vi "TEST - Delete Recursive (Read-Only).vi"(8 "error in (no error)":errorcluster) -> (0 "error out":errorcluster, 2 "pass":bool)   [LabVIEW 2020]
uses:
  source/library/File Exists/File Exists - Scalar.vi
  <userlib>/_OpenG.lib/error/error.llb/openg_error.lvlib
  source/library/openg_file.lvlib
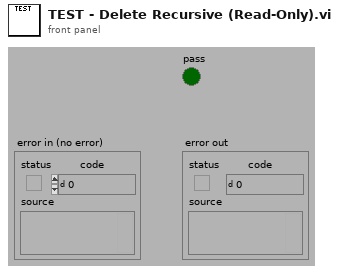
[diagram p1: front panel]
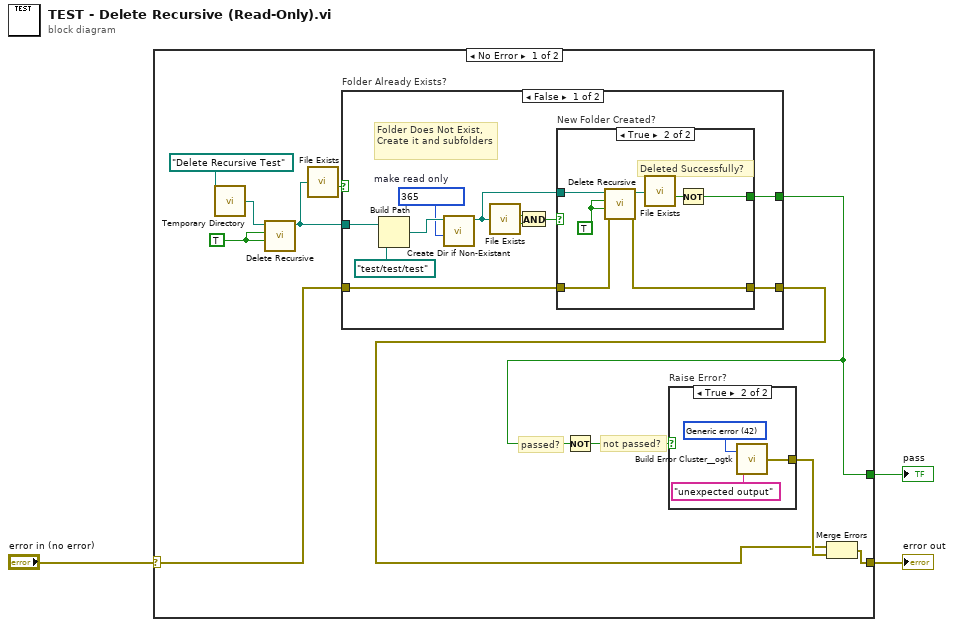
[diagram p0: block diagram]
diagram:
  n1 = case shown="No Error" "error in (no error)" {
    selector: "error in (no error)" -> [w4 w38]
    tunnel: [w5 _] -> w3
    tunnel: [w14 w38] -> w1
    frame No Error {
      w9 = TRUE ("Ignore Read-Only? (FALSE)")
      # "not passed?"
      # "passed?"
      n2 = call "Temporary Directory.vi"("Relative path (.)"=path "Delete Recursive Test") -> ("Temporary Directory (+ Relative)"=w10:path)
      n3 = call "Delete Recursive.vi"("Ignore Read-Only? (FALSE)"=w9, "Recursive? (FALSE)"=w9, "Path"=w10) -> ("dup Path"=w8:path)  [unwired: 7 in, 1 out]
      n4 = call-poly "File Exists.vi"("file path"=w8) -> ("exists"=w7:bool)  [unwired: 6 in, 1 out]
      n5 = case "Folder Already Exists?" shown="False" w7 {
        tunnel: w8 -> [w23 _]
        tunnel: [w18 w34] -> w6
        tunnel: [w17 _] -> w5
        tunnel: w4 -> [w16 w34]
        frame False {
          w15 = i16 365  # make read only
          # "Folder Does Not Exist, Create it and subfolders"
          n6 = Build Path(base path=w23, name or relative path=path "test/test/test" ("base path")) -> (appended path=w24:path)
          n7 = call "Create Dir if Non-Existant.vi"("permissions (0755)"=w15, "Directory Path"=w24) -> ("dup Directory Path"=w19:path)  [unwired: 7 in, 2 out]
          n8 = call-poly "File Exists.vi"("file path"=w19) -> ("is directory"=w22:bool, "exists"=w21:bool)  [unwired: 6 in]
          n9 = And(x=w22, y=w21) -> (x .and. y?=w20:bool)
          n10 = case "New Folder Created?" shown="True" w20 {
            tunnel: w19 -> [_ w33]
            tunnel: [w26 w31] -> w18
            tunnel: [_ w28] -> w17
            tunnel: w16 -> [w26 w27]
            frame False {
            }
            frame True {
              w32 = TRUE ("Recursive? (FALSE)")
              # "Deleted Successfully?"
              n11 = call "Delete Recursive.vi"("error in (no error)"=w27, "Ignore Read-Only? (FALSE)"=w32, "Recursive? (FALSE)"=w32, "Path"=w33) -> ("error out"=w31:errorcluster, "dup Path"=w30:path)  [unwired: 6 in]
              n12 = call-poly "File Exists.vi"("file path"=w30) -> ("exists"=w29:bool)  [unwired: 6 in, 1 out]
              n13 = Not(x=w29) -> (.not. x?=w28:bool)
            }
          }
        }
        frame True {
        }
      }
      n14 = Not(x=w5) -> (.not. x?=w12:bool)
      n15 = case "Raise Error?" shown="True" w12 {
        tunnel: [_ w35] -> w13
        frame False {
        }
        frame True {
          w36 = 42 items=["No error", "Argument error", "Memory is full", "Out of zone", "End of file", "File already open", "Generic file I/O error", "File not found", "File permission error", "Disk is full", "Duplicate path", "Too many files open", "System feature not enabled", "Resource file not found", "Cannot add resource", "Resource not found", "Image not found", "Image memory error", "Pen does not exist", "Config type invalid", "Config token not found", "Config parse error", "Config memory error", "Bad external code format", "Bad external code offset", "External code not present", "Null window", "Destroy window error", "Null menu", "Print aborted", "Bad print record", "Print driver error", "Windows error during printing", "Memory error during printing", "Print dialog error", "Generic print error", "Invalid device refnum", "Device not found", "Device parameter error", "Device unit error", "Cannot open device", "Device call aborted", "Generic error", "Cancelled by user", "Object ID too low", "Object ID too high", "Object not in heap", "Unknown heap", "Unknown object (invalid DefProc)", "Unknown object (DefProc not in table)", "Message out of range", "Invalid (null) method", "Unknown message", "Manager call not supported", "Bad address", "Network operation in progress", "Network operation timed out", "Connection is busy", "Network attribute not supported", "Network error", "Address in use", "System out of memory", "Connection aborted", "Connection refused", "Not connected", "Already connected", "Connection closed", "Initialization error (interapplication manager)", "Bad occurrence", "Wait on unbound occurrence handler", "Occurrence queue overflow", "Datalog type conflict", "Unused", "Unrecognized type (interapplication manager)", "Memory corrupt", "Failed to make temporary DLL", "Old CIN version", "Drag socket not found", "Failed to load drop-object", "Failed to register OLE object", "Failed to release OLE object", "Format specifier type mismatch", "Unknown format specifier", "Too few format specifiers", "Too many format specifiers", "Scan failed", "Newer CIN version", "Error converting to variant", "Runtime menu error", "Password tampered", "Variant attribute not found", "Incompatible variant data type", "Event data is not available", "Event Store is not present", "Occurrence is not found", "Event Queue is not created", "Event info is not available", "Refnum passed is NULL", "Error retrieving Class GUID", "Error retrieving CoClass GUID", "Error retrieving TypeLib GUID.", "Bad built application magic bytes.", "Specific driver is different from the specific driver associated with the Logical Name.", "There is no session opened to the class driver.", "Max Error", "MAX - Error with config objects", "MAX - Error loading configuration", "MAX - Group not supported"]
          n16 = call <userlib>:"Build Error Cluster__ogtk.vi"("String to Prepend to source (\"\")"="unexpected output" ("String to Prepend to source (\"\")"), "code"=w36) -> ("error out"=w35:errorcluster)
        }
      }
      n17 = Merge Errors(w6, w13) -> (w14:errorcluster)
    }
    frame Error {
    }
  }
  "pass" <- w3
  "error out" <- w1
